vi "Send Order to Handler.vi"(8 "error in (no error)":errorcluster, 10 "Order Out":refnum<class "Order.lvclass">, 11 "Customer In":refnum<class "Customer.lvclass">) -> (0 "error out":errorcluster, 3 "Customer Out":refnum<class "Customer.lvclass">)   [LabVIEW 2020, in "Customer.lvclass"]
uses:
  Customer.lvclass
  Support/Order/Order.lvclass
  Customer.lvclass/Customer.ctl
  Process Job/Job Handler.lvclass
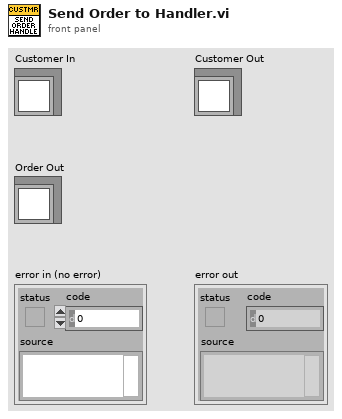
[diagram p1: front panel]
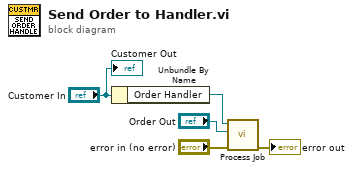
[diagram p0: block diagram]
diagram:
  n1 = Unbundle By Name("Customer In") -> ("Order Handler"=w4:refnum<class "Job Handler.lvclass">)
  n2 = call-dynamic "Process Job.vi"("error in (no error)"="error in (no error)", "Job"="Order Out", "Process Job In"=w4) -> ("error out"=→"error out":errorcluster)  [unwired: 7 in, 1 out]
  "Customer Out" <- "Customer In"
